vi "Set ENUM Properties.vi"(8 "error in":errorcluster, 10 "enum to be changes":T1(array[cluster]), 11 "parent ref in":T2 format="%.0x") -> (0 "error out":errorcluster, 3 "parent ref out":T2 format="%.0x")   [LabVIEW 2020, in "AIM ARINC 664 Scripting.lvlib"]
uses:
  AIM ARINC 664 Scripting.lvlib
  <vilib>/NI VeriStand/Custom Device API/Custom Device Item Ref.ctl
  <vilib>/NI VeriStand/Custom Device Tools/Custom Device Utility Library/NI VeriStand - Search for Item by Name.vi
  <vilib>/NI VeriStand/Custom Device Tools/Custom Device Utility Library/Custom Device Utility Library.lvlib
  <vilib>/NI/NI VeriStand Advanced SysDef API/SysDef API/Advanced System Definition.lvlib
  <vilib>/NI VeriStand/Custom Device API/Custom Device API.lvlib
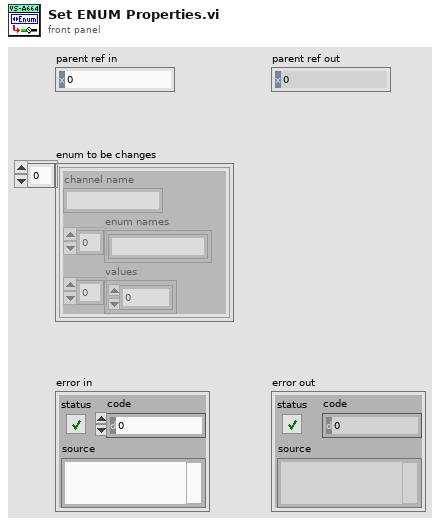
[diagram p1: front panel]
types:
  T1 = cluster{"channel name":string, "enum names":string[], "values":dbl[]}[]
  T2 = typedef "Custom Device API.lvlib/Custom Device Item Ref.ctl" = u64
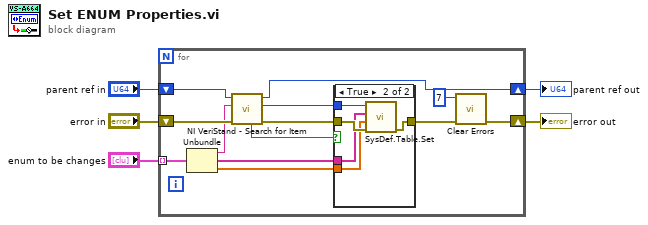
[diagram p0: block diagram]
diagram:
  n1 = for {
    shift-right: [w7] -> w2
    shift-left: "error in" -> [w17]
    tunnel: "enum to be changes" -> [w13] mode=indexing
    shift-right: [w8] -> w5
    shift-left: "parent ref in" -> [w18]
    n2 = Unbundle(w13) -> ("channel name"=w12:string, "enum names"=w11:string[], "values"=w10:dbl[])
    n3 = call-poly <vilib>:"NI VeriStand - Search for Item.vi"("error in"=w17, "Item Name"=w12, "Section Ref in"=w18) -> ("error out"=w15:errorcluster, "Item Ref"=w9:T2, "Section Ref out"=w8:T2, "Found"=w16:bool)  [unwired: 5 in]
    n4 = case shown="True" w16 {
      tunnel: w15 -> [w19 w24]
      tunnel: [w19 w23] -> w14
      tunnel: w11 -> [_ w22]
      tunnel: w10 -> [_ w21]
      tunnel: w9 -> [_ w20]
      frame False {
      }
      frame True {
        n5 = call <vilib>:"SysDef.Table.Set.vi"("error in (no error)"=w24, "Values"=w21, "Names"=w22, "nodeID"=w20) -> ("error out"=w23:errorcluster)  [unwired: 6 in, 1 out]
      }
    }
    n6 = call <vilib>:"Clear Errors.vi"("error in (no error)"=w14, "specific error code to clear (0: all)"=7) -> ("error out"=w7:errorcluster)  [unwired: 4 in, 1 out]
  }
  "parent ref out" <- w5
  "error out" <- w2
